vi "INI_bk9132b.vi"(5 "MCListbox Ref":refnum<vi>, 9 "MCList Box Row":u8=3 max=8, 11 "Device INI Config File Path":path=path "D:/LABVIEW/Examples/INI Devices/DeviceConfig.ini") -> (0 "error out":errorcluster, 3 "Serial_VISA":T1)   [LabVIEW 2018]
uses:
  Examples - 32bit/SEQUENCER/SEQUENSER v10/Sequencer v10/Ctl/Serial_VISA.ctl
  <vilib>/Utility/miscctls.llb/LVRowAndColumnTypeDef.ctl
  <vilib>/Utility/config.llb/Read Key (String).vi
  <vilib>/Utility/config.llb/NI_LVConfig.lvlib
  <instrlib>/BK Precision 913XX/BK Precision 913XX.lvlib
panel:
  out "PowSupplay array":string[](array[string])
  out "PowSupply Read Buffer":string
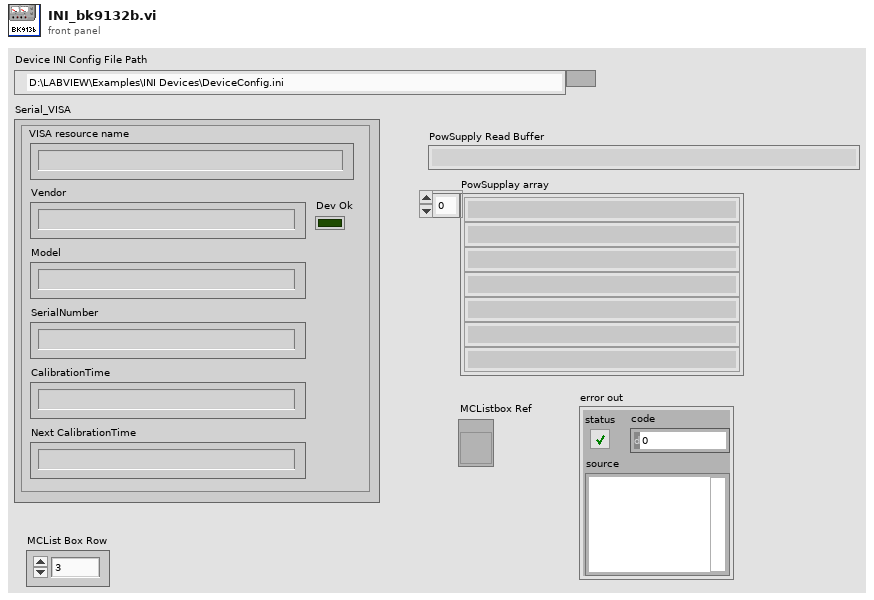
[diagram p1: front panel]
types:
  T1 = typedef "Serial_VISA.ctl" = cluster{"VISA resource name":string, "Vendor":string, "SerialNumber":string, "CalibrationTime":string, "Dev Ok":bool, "Model":string, "Next CalibrationTime":string}
  T2 = typedef "LVRowAndColumnTypeDef.ctl" = cluster{"Row":i32, "Column":i32}
  T3 = typedef "NI_LVConfig.lvlib/Config Data RefNum.ctl" = refnum<k1>
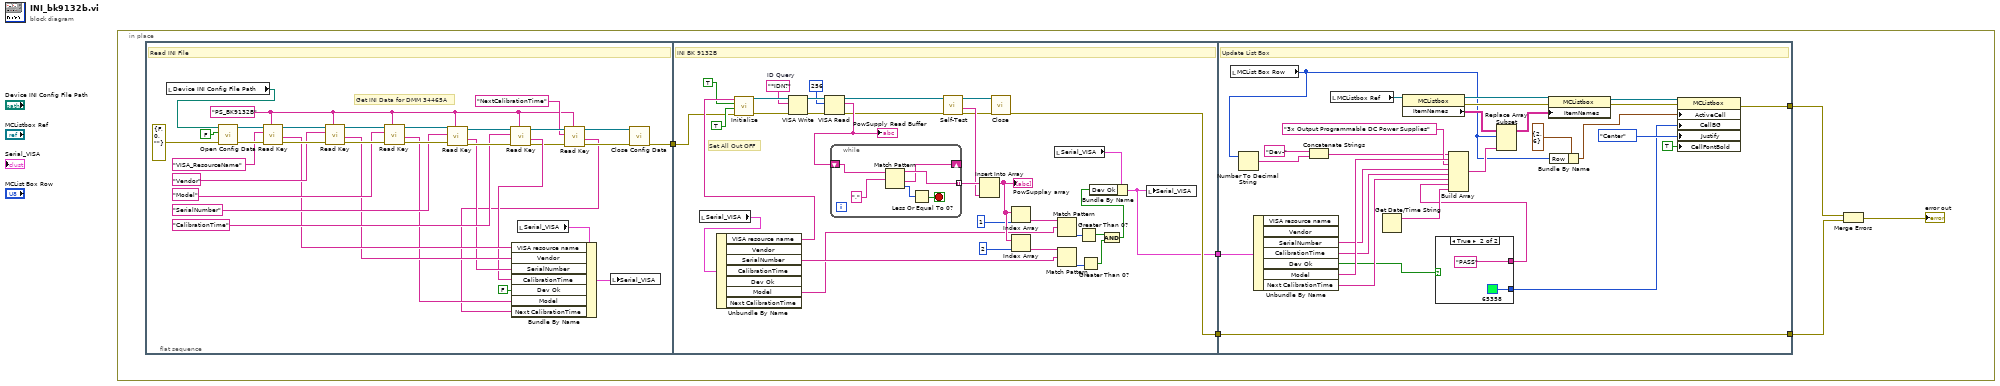
[diagram p0: block diagram]
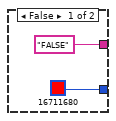
[diagram p2: hidden frame]
diagram:
  n1 = in-place {
    n2 = flat-sequence {
      tunnel: [w9] -> w6
      tunnel: w6 -> [w43]
      tunnel: [w42] -> w4
      tunnel: [w41] -> w1
      tunnel: [w87] -> w5
      tunnel: [w86] -> w3
      tunnel: w4 -> [w86]
      tunnel: w1 -> [w84]
      frame #0 {
        w13 = "PS_BK9132B" ("section")
        # "Get INI Data for DMM 34465A"
        # "Read INI File"
        n3 = local read "Device INI Config File Path"() -> (w11:path)
        n4 = call <vilib>:"Open Config Data.vi"("error in (no error)"=errorcluster {"status"=FALSE, "code"=0, "source"=""} ("error constant"), "create file if necessary (T)"=FALSE, "configuration file path"=w11) -> ("error out"=w38:errorcluster, "refnum"=w39:T3)  [unwired: 6 in, 1 out]
        n5 = call-poly <vilib>:"Read Key.vi"("section"=w13, "error in (no error)"=w38, "key"="VISA_ResourceName", "refnum"=w39) -> ("error out"=w35:errorcluster, "value"=w24:string, "refnum out"=w37:T3)  [unwired: 4 in, 1 out]
        n6 = call-poly <vilib>:"Read Key.vi"("section"=w13, "error in (no error)"=w35, "key"="Vendor", "refnum"=w37) -> ("error out"=w34:errorcluster, "value"=w23:string, "refnum out"=w36:T3)  [unwired: 4 in, 1 out]
        n7 = call-poly <vilib>:"Read Key.vi"("section"=w13, "error in (no error)"=w34, "key"="Model", "refnum"=w36) -> ("error out"=w29:errorcluster, "value"=w22:string, "refnum out"=w30:T3)  [unwired: 4 in, 1 out]
        n8 = call-poly <vilib>:"Read Key.vi"("section"=w13, "error in (no error)"=w29, "key"="SerialNumber", "refnum"=w30) -> ("error out"=w26:errorcluster, "value"=w21:string, "refnum out"=w27:T3)  [unwired: 4 in, 1 out]
        n9 = call-poly <vilib>:"Read Key.vi"("section"=w13, "error in (no error)"=w26, "key"="CalibrationTime", "refnum"=w27) -> ("error out"=w17:errorcluster, "value"=w20:string, "refnum out"=w18:T3)  [unwired: 4 in, 1 out]
        n10 = local read "Serial_VISA"() -> (w8:T1)
        n11 = call-poly <vilib>:"Read Key.vi"("section"=w13, "error in (no error)"=w17, "key"="NextCalibrationTime", "refnum"=w18) -> ("error out"=w15:errorcluster, "value"=w12:string, "refnum out"=w16:T3)  [unwired: 4 in, 1 out]
        n12 = Bundle By Name(cluster=w8, "VISA resource name"=w24, "Vendor"=w23, "SerialNumber"=w21, "CalibrationTime"=w20, "Dev Ok"=FALSE, "Model"=w22, "Next CalibrationTime"=w12) -> (w7:T1)
        n13 = local write "Serial_VISA"(w7) -> ()
        n14 = call <vilib>:"Close Config Data.vi"("error in (no error)"=w15, "refnum"=w16) -> ("error out"=w9:errorcluster)  [unwired: 8 in, 1 out]
      }
      frame #1 {
        w48 = "*IDN?"  # ID Query
        # "Set All Out OFF"
        # "INI BK 9132B"
        n15 = local read "Serial_VISA"() -> (w45:T1)
        n16 = Unbundle By Name(w45) -> ("VISA resource name"=w52:string, "SerialNumber"=w67:string, "Model"=w65:string)  [unwired: 4 out]
        n17 = call <instrlib>:"Initialize.vi"("error in (no error)"=w43, "Reset (True)"=TRUE, "ID Query (True)"=TRUE, "VISA resource name"=w52) -> ("error out"=w56:errorcluster, "VISA resource name out"=w55:refnum<visa-resource-name>)  [unwired: 6 in]
        n18 = VISA Write(VISA resource name=w55, write buffer=w48, error in (no error)=w56) -> (VISA resource name out=w53:refnum<visa-resource-name>, error out=w54:errorcluster)  [unwired: 1 out]
        n19 = VISA Read(VISA resource name=w53, byte count=u32 256, error in (no error)=w54) -> (VISA resource name out=w57:refnum<visa-resource-name>, read buffer=w62:string, error out=w58:errorcluster)  [unwired: 1 out]
        "PowSupply Read Buffer" <- w62
        n20 = while {
          shift-right: [w76] -> _
          shift-left: w62 -> [w79]
          tunnel: [w77] -> w63 mode=indexing
          stop <- w74 stop-if-true
          n21 = Match Pattern(string=w79, regular expression="," ("search string/char (-)")) -> (before substring=w77:string, after substring=w76:string, offset past match=w75:i32)  [unwired: 1 in, 1 out]
          n22 = Less Or Equal To 0?(x=w75) -> (x <= 0?=w74:bool)
        }
        n23 = call <instrlib>:"Self-Test.vi"("error in (no error)"=w58, "VISA resource name"=w57) -> ("error out"=w59:errorcluster, "Self-Test Result Message"=w61:string, "VISA resource name out"=w60:refnum<visa-resource-name>)  [unwired: 6 in, 1 out]
        n24 = Insert Into Array(array=w63, new element=w61) -> (w72:string[])  [unwired: 1 in]
        "PowSupplay array" <- w72
        n25 = call <instrlib>:"Close.vi"("error in (no error)"=w59, "VISA resource name"=w60) -> ("error out"=w42:errorcluster)  [unwired: 9 in]
        n26 = Index Array(array=w72, index=1) -> (element=w64:string)
        n27 = Index Array(array=w72, index=2) -> (element=w66:string)
        n28 = local read "Serial_VISA"() -> (w44:T1)
        n29 = Match Pattern(string=w64, regular expression=w65) -> (offset past match=w68:i32)  [unwired: 1 in, 3 out]
        n30 = Match Pattern(string=w66, regular expression=w67) -> (offset past match=w70:i32)  [unwired: 1 in, 3 out]
        n31 = Greater Than 0?(x=w68) -> (x > 0?=w69:bool)
        n32 = Greater Than 0?(x=w70) -> (x > 0?=w71:bool)
        n33 = And(x=w69, y=w71) -> (x .and. y?=w73:bool)
        n34 = Bundle By Name(cluster=w44, "Dev Ok"=w73) -> (w41:T1)
        n35 = local write "Serial_VISA"(w41) -> ()
      }
      frame #2 {
        # "Update List Box"
        n36 = local read "MCList Box Row"() -> (w83:u8)
        n37 = Number To Decimal String(number=w83) -> (decimal integer string=w81:string)  [unwired: 1 in]
        n38 = Unbundle By Name(w84) -> ("SerialNumber"=w104:string, "CalibrationTime"=w105:string, "Dev Ok"=w90:bool, "Model"=w106:string, "Next CalibrationTime"=w107:string)  [unwired: 2 out]
        n39 = Concatenate Strings("Dev-", w81) -> (w80:string)
        n40 = local read "MCListbox Ref"() -> (w94:refnum<vi>)
        n41 = Get Date/Time String() -> (date string=w93:string)  [unwired: 3 in, 1 out]
        n42 = property class="MCListbox"(reference=w94) -> (reference out=w97:refnum<vi>, error out=w98:errorcluster, "ItemNames"=w99:string[][])  [unwired: 1 in]
        n43 = case shown="True" w90 {
          tunnel: [u32 16711680 u32 65358] -> w89
          tunnel: ["FALSE" ("element") "PASS" ("element")] -> w88
          frame False {
          }
          frame True {
          }
        }
        n44 = Build Array(w80, w106, "3x Output Programmable DC Power Supplies", w104, w105, w107, w88, w93) -> (w101:string[])
        n45 = Replace Array Subset(array=w99, new element=w101, index (row)=w83) -> (w100:string[][])  [unwired: 1 in]
        n46 = property class="MCListbox"(reference=w97, error in=w98, "ItemNames"=w100) -> (reference out=w102:refnum<vi>, error out=w103:errorcluster)
        n47 = Bundle By Name(cluster=T2 {"Row"=2, "Column"=6} ("Active Cell:Active Cell"), "Row"=w83) -> (w91:T2)
        n48 = property class="MCListbox"(reference=w102, error in=w103, "ActiveCell"=w91, "CellBG"=w89, "Justify"=enum16{"Left", "Center", "Right"}."Center" ("Active Cell:Cell Justification"), "CellFontBold"=TRUE ("Active Cell:Cell Font:Bold")) -> (error out=w87:errorcluster)  [unwired: 1 out]
      }
    }
    n49 = Merge Errors(w5, w3) -> (→"error out":errorcluster)
  }
